vi "DAQFIFO_HH.vi"(0 "mode":u16(ring) items=["standalone", "dialog"]) -> ()   [LabVIEW 2009]
panel:
  in  "rebinning":dbl=16.0
  in  ".sm file format":bool
  in  "Exit":bool caption="stop"
  in  "Show Decay":bool=TRUE
  out "Counts":cluster{"Total":u32, "Gap":u32, "Invalid":u32}
  in  "Save & Exit":bool caption="stop"
  in  "Run":bool
  out "MCS":i32[][](graph)
  in  "Destination:":path
  in  "Store Data":bool caption="Store Data:"
  out "Decay":cluster{dbl[], u32[]}[](graph)
  out "SPC_rates":T1={"SYNC"=9999872.0, "Ch1"=44672.0, "Ch2"=44496.0, "Ch3"=44496.0, "Ch4"=44496.0, "Sync LED"=FALSE} {"Ch4" scale=1000.0..100000.0 scale format="%.0e"; "Ch3" scale=1000.0..100000.0 scale format="%.0e"; "Ch2" scale=1000.0..100000.0 scale format="%.0e"; "Ch1" min=0.0 max=8000000.0 scale=1.0..100000.0 scale format="%.0e"; "SYNC" min=0.0 max=100000000.0 scale=100000.0..100000000.0 scale format="%.0e"}
  in  "Tab Control":T2(tab)
  in  "Measurement":T3={"Binning (ms)"=1.0, "External Trigger Condition?"=0, "Stop Condition:"=2, "Stop Count"=120.0, "Buffer Size (Photons)?"=36864, "No of Channels?"=7, "Ext Latch Delay?"=0} {"Ext Latch Delay?" min=0 max=255 step=1; "Buffer Size (Photons)?" min=512 max=131072 step=512; "Stop Count" format="%.2f"; "Stop Condition:" items=["None", "Photon Count", "Time (s)"]; "No of Channels?" max=255 step=1; "Binning (ms)" min=1e-07 max=100000 format="%.3f"}
  in  "ADC":T4={"Binning (HH)"=1, "?Dither Range"=0, "?Count Increment"=1, "Mode"=1} {"Mode" items=["T3"]; "Binning (HH)" items=["1", "2", "4", "8", "16", "32", "64", "128", "256", "512", "1024"]; "?Count Increment" min=1 max=255 step=1; "?Dither Range" min=0 max=256 step=32}
  in  "SYNC":T5={"SYNC ZC Level (mV)"=10.0, "SYNC Freq Divider"=3, "SYNC Holdoff (ps)"=0.0, "SYNC Threshold (mV)"=200.0} {"SYNC Threshold (mV)" min=0 max=1000 format="%.2f"; "SYNC Holdoff (ps)" min=-99999 max=99999 format="%.2f"; "SYNC Freq Divider" items=["1", "2", "4", "8", "16"]; "SYNC ZC Level (mV)" min=0 max=40 format="%.2f"}
  in  "Ch1":T6={"Ch1 ZC Level (mV)"=10.0, "Ch1 Holdoff (ps)"=0.0, "Ch1 Threshold (mV)"=200.0} {"Ch1 Threshold (mV)" min=0 max=1000 format="%.2f"; "Ch1 Holdoff (ps)" min=-99999 max=99999 format="%.2f"; "Ch1 ZC Level (mV)" min=0 max=40 format="%.2f"}
  in  "Ch 2":T7={"Ch2 ZC Level (mV)"=10.0, "Ch2 Holdoff (ps)"=0.0, "Ch2 Threshold (mV)"=200.0} {"Ch2 Threshold (mV)" min=0 max=1000 format="%.2f"; "Ch2 Holdoff (ps)" min=-99999 max=99999 format="%.2f"; "Ch2 ZC Level (mV)" min=0 max=40 format="%.2f"}
  in  "Ch 3":T8={"Ch3 ZC Level (mV)"=10.0, "Ch3 Holdoff (ps)"=0.0, "Ch3 Threshold (mV)"=200.0} {"Ch3 Threshold (mV)" min=0 max=1000 format="%.2f"; "Ch3 Holdoff (ps)" min=-99999 max=99999 format="%.2f"; "Ch3 ZC Level (mV)" min=0 max=40 format="%.2f"}
  in  "Ch 4":T9={"Ch4 ZC Level (mV)"=10.0, "Ch4 Holdoff (ps)"=0.0, "Ch4 Threshold (mV)"=200.0} {"Ch4 Threshold (mV)" min=0 max=1000 format="%.2f"; "Ch4 Holdoff (ps)" min=-99999 max=99999 format="%.2f"; "Ch4 ZC Level (mV)" min=0 max=40 format="%.2f"}
  in  "TAC":T10={"TAC Range [ns]"=50.0, "TAC Gain"=2, "TAC Offset [%]"=0.0, "TAC Limit Low [%]"=0.0, "TAC Limit High [%]"=100.0} {"TAC Limit High [%]" min=0 max=100 format="%.2f"; "TAC Limit Low [%]" min=0 max=100 format="%.2f"; "TAC Offset [%]" min=0 max=100 format="%.2f"; "TAC Gain" min=1 max=15 step=1; "TAC Range [ns]" min=0 max=2000 format="%.2f"}
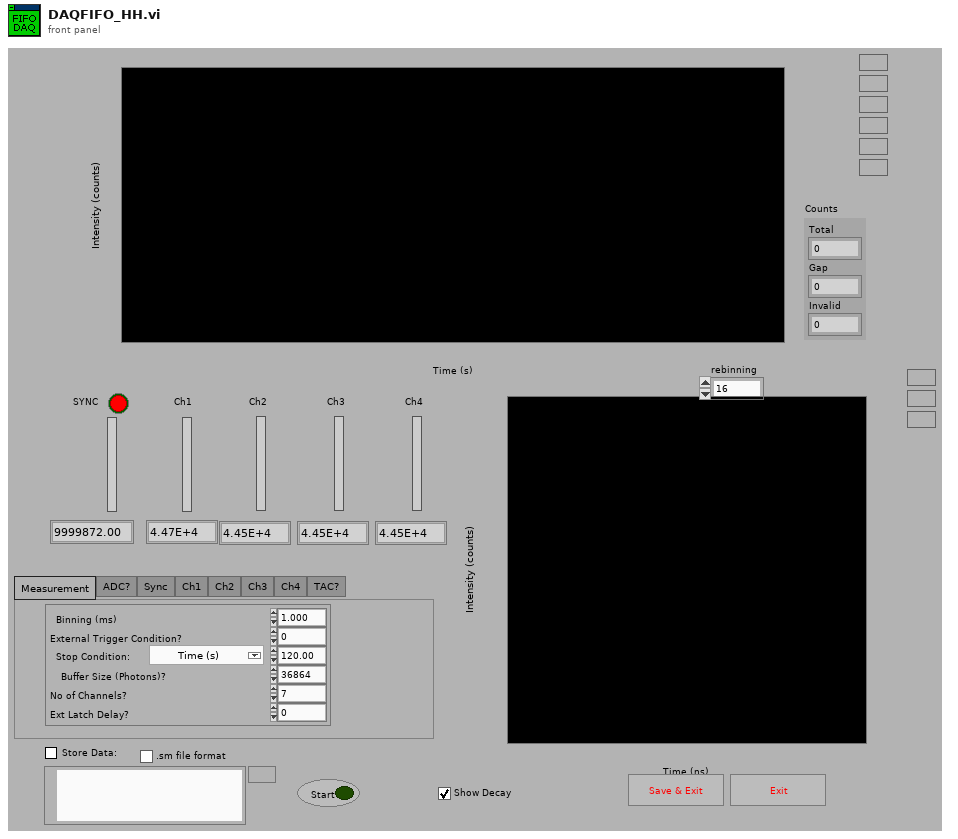
[diagram p1: front panel]
types:
  T1 = cluster{"SYNC":dbl, "Ch1":dbl, "Ch2":dbl, "Ch3":dbl, "Ch4":dbl, "Sync LED":bool}
  T2 = enum32{"Measurement", "ADC?", "Sync", "Ch1", "Ch2", "Ch3", "Ch4", "TAC?"}
  T3 = cluster{"Binning (ms)":sgl, "External Trigger Condition?":u16, "Stop Condition:":u16, "Stop Count":dbl, "Buffer Size (Photons)?":u32, "No of Channels?":u16, "Ext Latch Delay?":i16}
  T4 = cluster{"Binning (HH)":i16, "?Dither Range":i16, "?Count Increment":i16, "Mode":u16}
  T5 = cluster{"SYNC ZC Level (mV)":sgl, "SYNC Freq Divider":u16, "SYNC Holdoff (ps)":sgl, "SYNC Threshold (mV)":sgl}
  T6 = cluster{"Ch1 ZC Level (mV)":sgl, "Ch1 Holdoff (ps)":sgl, "Ch1 Threshold (mV)":sgl}
  T7 = cluster{"Ch2 ZC Level (mV)":sgl, "Ch2 Holdoff (ps)":sgl, "Ch2 Threshold (mV)":sgl}
  T8 = cluster{"Ch3 ZC Level (mV)":sgl, "Ch3 Holdoff (ps)":sgl, "Ch3 Threshold (mV)":sgl}
  T9 = cluster{"Ch4 ZC Level (mV)":sgl, "Ch4 Holdoff (ps)":sgl, "Ch4 Threshold (mV)":sgl}
  T10 = cluster{"TAC Range [ns]":sgl, "TAC Gain":i16, "TAC Offset [%]":sgl, "TAC Limit Low [%]":sgl, "TAC Limit High [%]":sgl}
  T11 = typedef "FIFOSettings.ctt" = cluster{"Measurement":cluster{"Binning (ms)":sgl, "External Trigger Condition":u16, "Stop Condition:":u16, "Stop Count":dbl, "Buffer Size (Photons)":u32, "No of Channels":u16, "Ext Latch Delay":i16}, "ADC":cluster{"Binning (HH)":i16, "Dither Range":i16, "Count Increment":i16, "Mode":u16}, "SYNC":cluster{"SYNC ZC Level (mV)":sgl, "SYNC Freq Divider":u16, "SYNC Holdoff (ps)":sgl, "SYNC Threshold (mV)":sgl}, "TAC":cluster{"TAC Range (ns)":sgl, "TAC Gain":i16, "TAC Offset (%)":sgl, "TAC Limit Low (%)":sgl, "TAC Limit High (%)":sgl}, "Ch 2":cluster{"Ch2 ZC Level (mV)":sgl, "Ch2 Holdoff (ps)":sgl, "Ch2 Threshold (mV)":sgl}, "Ch 3":cluster{"Ch3 ZC Level (mV)":sgl, "Ch3 Holdoff (ps)":sgl, "Ch3 Threshold (mV)":sgl}, "Ch 4":cluster{"Ch4 ZC Level (mV)":sgl, "Ch4 Holdoff (ps)":sgl, "Ch4 Threshold (mV)":sgl}, "Ch1":cluster{"Ch1 ZC Level (mV)":sgl, "Ch1 Holdoff (ps)":sgl, "Ch1 Threshold (mV)":sgl}}
  T12 = cluster{"Binning (ms)":sgl, "External Trigger Condition":u16, "Stop Condition:":u16, "Stop Count":dbl, "Buffer Size (Photons)":u32, "No of Channels":u16, "Ext Latch Delay":i16}
  T13 = cluster{"Binning (HH)":i16, "Dither Range":i16, "Count Increment":i16, "Mode":u16}
  T14 = cluster{"TAC Range (ns)":sgl, "TAC Gain":i16, "TAC Offset (%)":sgl, "TAC Limit Low (%)":sgl, "TAC Limit High (%)":sgl}
  T15 = cluster{"router channels":u8[], "macro times(50ns steps)":u32[], "micro times":u16[], "invalid times":u32[], "gap times":u32[]}
  T16 = cluster{"Sync_rate":sgl, "Ch1":sgl, "Ch2":sgl, "Ch3":sgl, "Ch 4":sgl, "Sync":bool}
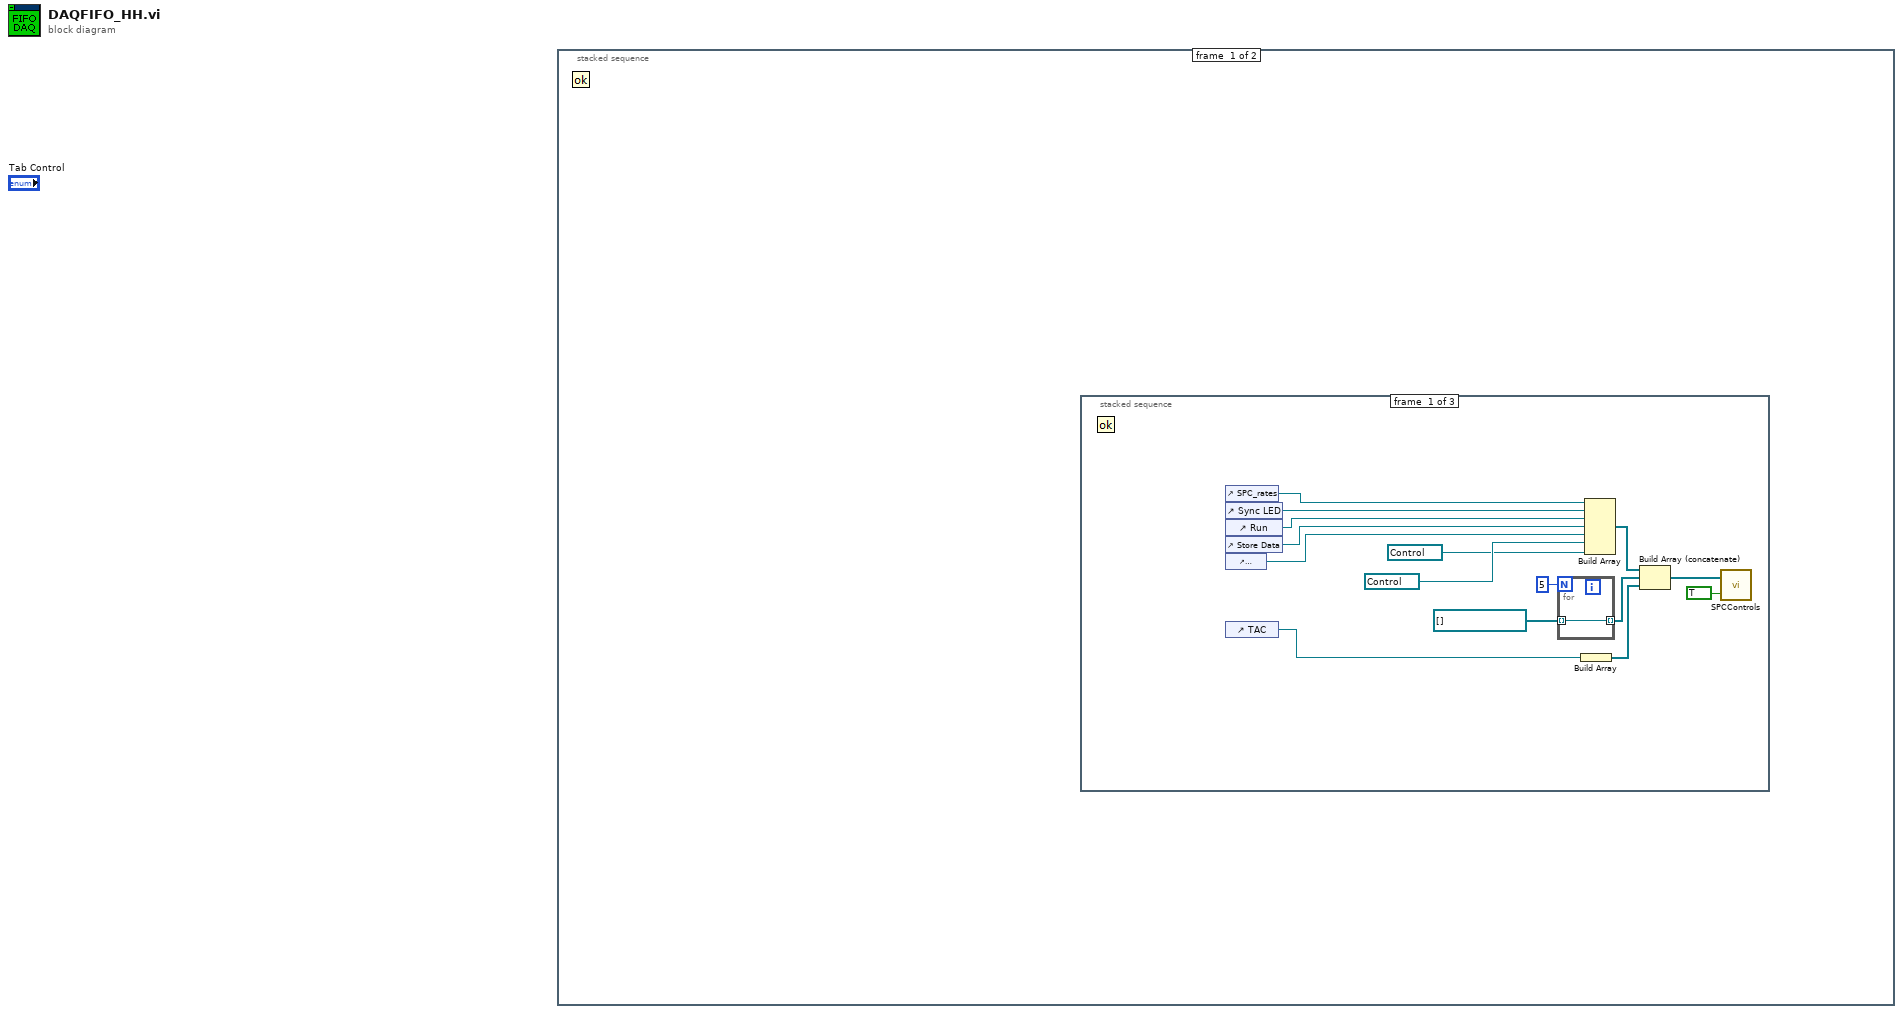
[diagram p0: block diagram]
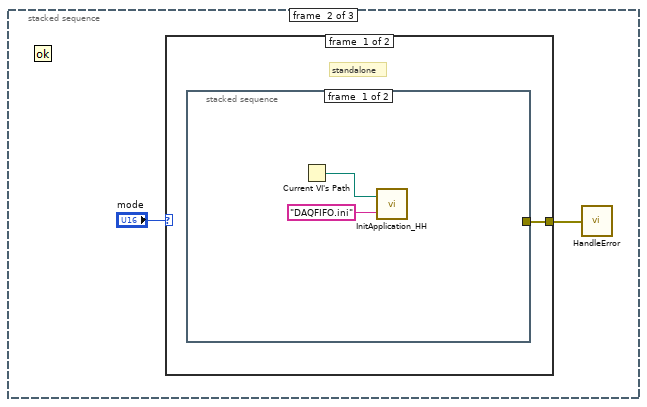
[diagram p2: hidden frame]
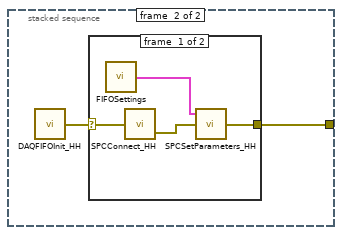
[diagram p3: hidden frame]
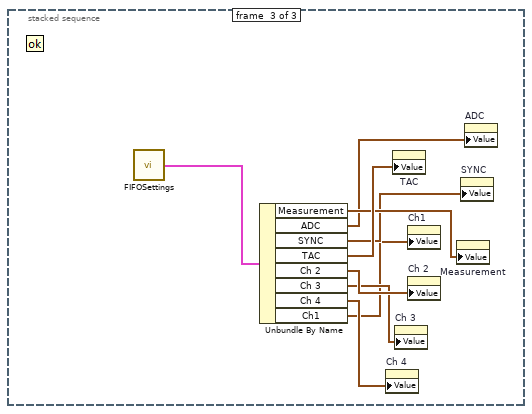
[diagram p6: hidden frame]
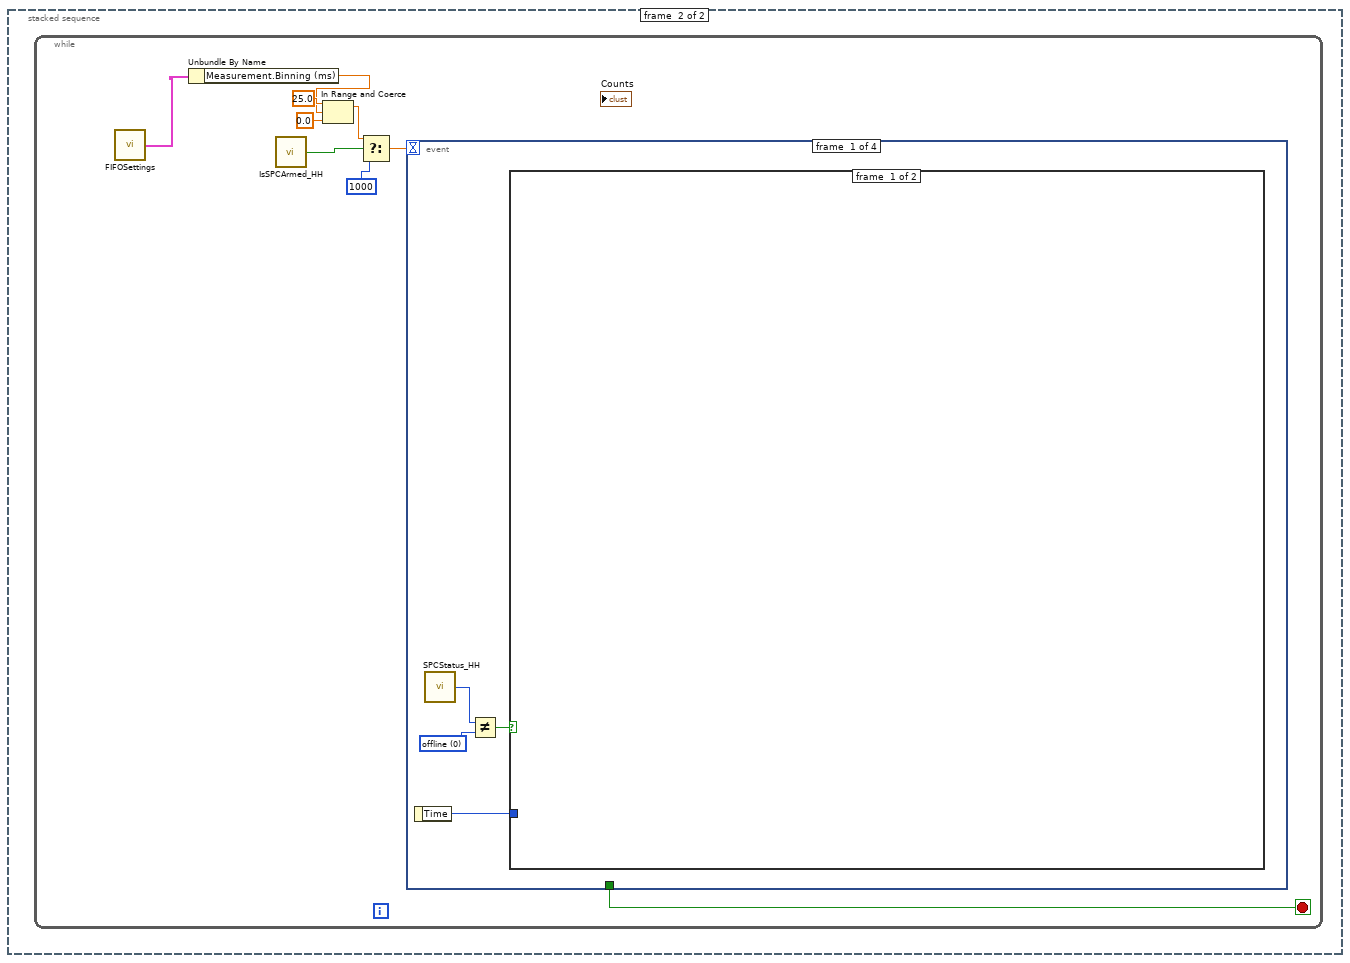
[diagram p7: hidden frame]
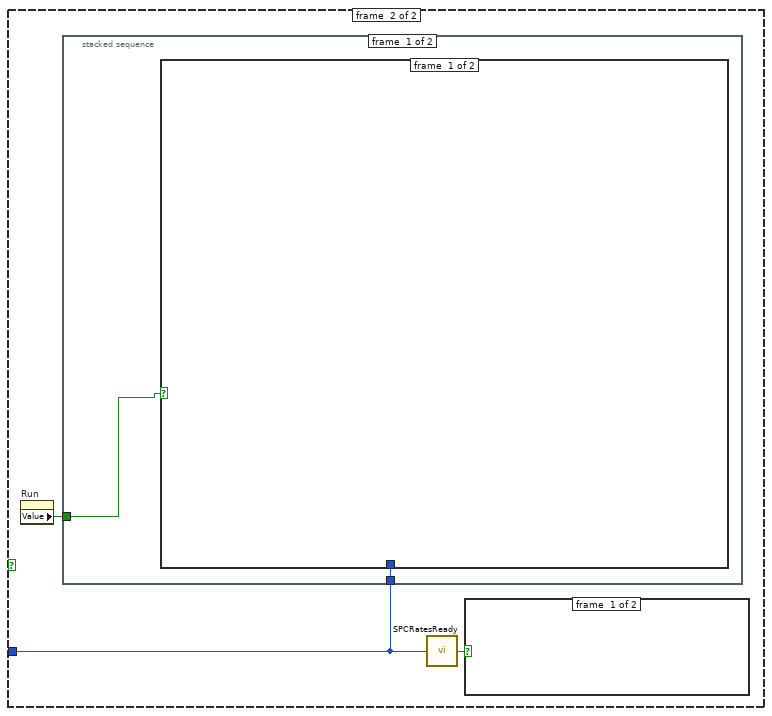
[diagram p8: hidden frame]
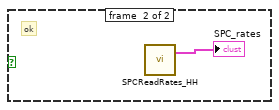
[diagram p9: hidden frame]
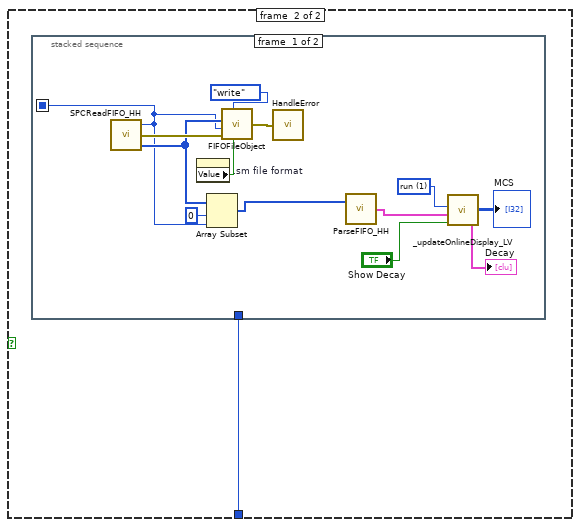
[diagram p10: hidden frame]
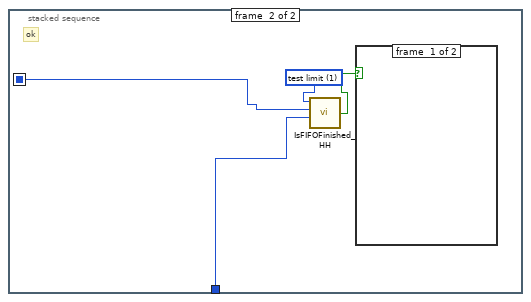
[diagram p11: hidden frame]
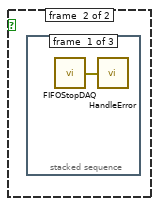
[diagram p12: hidden frame]
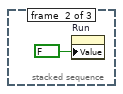
[diagram p13: hidden frame]
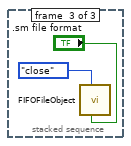
[diagram p14: hidden frame]
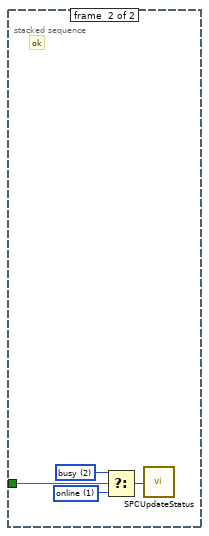
[diagram p15: hidden frame]
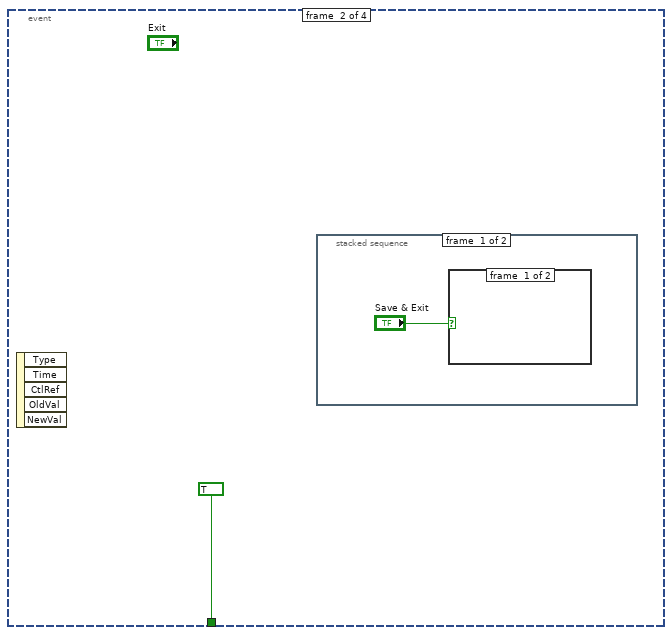
[diagram p16: hidden frame]
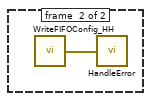
[diagram p17: hidden frame]
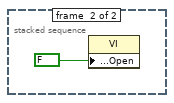
[diagram p18: hidden frame]
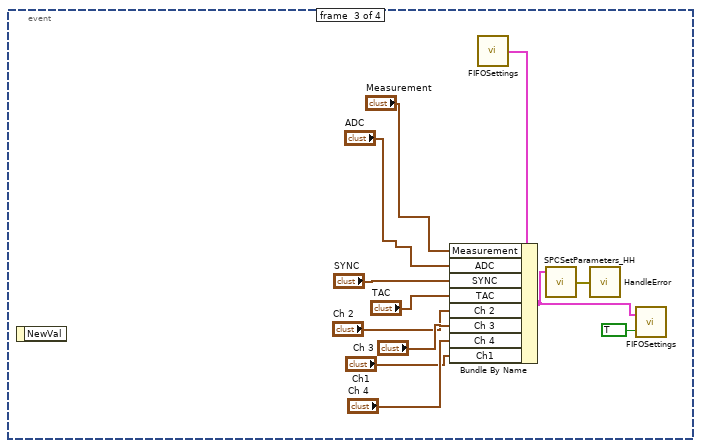
[diagram p19: hidden frame]
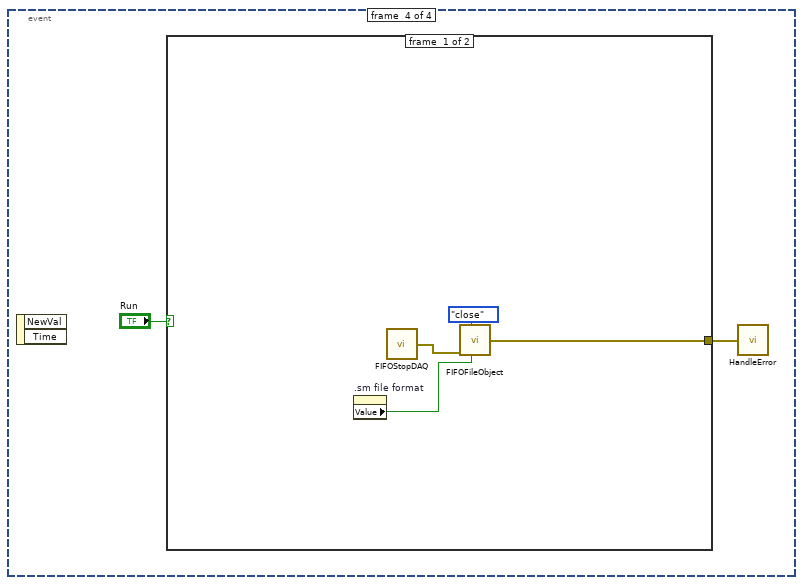
[diagram p20: hidden frame]
diagram:
  n1 = stacked-sequence {
    frame #0 {
      n2 = stacked-sequence {
        frame #0 {
          n3 = control-ref of="SPC_rates"() -> (w14:refnum<vi>)
          n4 = control-ref of="Sync LED"() -> (w13:refnum<vi>)
          n5 = control-ref of="Run"() -> (w8:refnum<vi>)
          n6 = control-ref of="Store Data"() -> (w9:refnum<vi>)
          n7 = control-ref of="Destination:"() -> (w10:refnum<vi>)
          n8 = control-ref of="TAC"() -> (w15:refnum<vi>)
          n9 = for {
            N: 5 -> [_]
            tunnel: refnum<vi>[] [] ("Controls[]") -> [w16] mode=indexing
            tunnel: [w16] -> w4 mode=indexing
          }
          n10 = Build Array(w15) -> (w12:refnum<vi>[])
          n11 = Build Array(w14, w13, w8, w9, w10, refnum<vi> refnum ("Element"), refnum<vi> refnum ("Element")) -> (w11:refnum<vi>[])
          n12 = Build Array (concatenate)(w11, w4, w12) -> (w7:refnum<vi>[])
          n13 = call "SPCControls.vi"("Set/Get"=TRUE, "Control References (input)"=w7) -> ()  [unwired: 1 out]
        }
        frame #1 {
          n14 = case shown="0, Default" "mode" {
            tunnel: [w19 _] -> w17
            frame #0 {
              # "standalone"
              n15 = stacked-sequence {
                tunnel: [_ w22] -> w19
                frame #0 {
                  n16 = Current VI's Path() -> (path=w21:path)
                  n17 = call "InitApplication_HH.vi"("file name"="DAQFIFO.ini" ("configuration file path"), "VI path"=w21) -> ()
                }
                frame #1 {
                  n18 = call "DAQFIFOInit_HH.vi"() -> ("error out"=w23:errorcluster)  [unwired: 1 in]
                  n19 = case shown="No Error" w23 {
                    selector: w23 -> [w27 w28]
                    tunnel: [w25 w28] -> w22
                    frame #0 {
                      n20 = call "FIFOSettings.vi"() -> ("FIFO Settings(out)"=w24:T11)  [unwired: 2 in]
                      n21 = call "SPCConnect_HH.vi"("error in (no error)"=w27) -> ("Error out"=w26:errorcluster)  [unwired: 1 in]
                      n22 = call "SPCSetParameters_HH.vi"("error in (no error)"=w26, "FIFO Settings"=w24) -> ("error (out)"=w25:errorcluster)  [unwired: 1 in]
                    }
                    frame #1 {
                    }
                  }
                }
              }
            }
            frame #1 {
              # "dialog"
            }
          }
          n23 = call "HandleError.vi"("error in (no error)"=w17) -> ()
        }
        frame #2 {
          n24 = call "FIFOSettings.vi"() -> ("FIFO Settings(out)"=w29:T11)  [unwired: 2 in]
          n25 = Unbundle By Name(w29) -> ("Measurement"=w36:T12, "ADC"=w35:T13, "SYNC"=w34:T5, "TAC"=w37:T14, "Ch 2"=w33:T7, "Ch 3"=w32:T8, "Ch 4"=w31:T9, "Ch1"=w30:T6)
          n26 = property on="Ch 4" class="Cluster (strikt)"("Value"=w31) -> ()  [unwired: 2 in, 2 out]
          n27 = property on="TAC" class="Cluster (strict)"("Value"=w37) -> ()  [unwired: 2 in, 2 out]
          n28 = property on="Ch 3" class="Cluster (strikt)"("Value"=w32) -> ()  [unwired: 2 in, 2 out]
          n29 = property on="Ch1" class="Cluster (strikt)"("Value"=w30) -> ()  [unwired: 2 in, 2 out]
          n30 = property on="Ch 2" class="Cluster (strikt)"("Value"=w33) -> ()  [unwired: 2 in, 2 out]
          n31 = property on="Measurement" class="Cluster (strikt)"("Value"=w36) -> ()  [unwired: 2 in, 2 out]
          n32 = property on="SYNC" class="Cluster (strikt)"("Value"=w34) -> ()  [unwired: 2 in, 2 out]
          n33 = property on="ADC" class="Cluster (strikt)"("Value"=w35) -> ()  [unwired: 2 in, 2 out]
        }
      }
    }
    frame #1 {
      n34 = while {
        stop <- w43 stop-if-true
        n35 = call "FIFOSettings.vi"() -> ("FIFO Settings(out)"=w38:T11)  [unwired: 2 in]
        n36 = Unbundle By Name(w38) -> ("Measurement.Binning (ms)"=w40:sgl)
        n37 = call "IsSPCArmed_HH.vi"() -> ("Boolean"=w46:bool)  [unwired: 1 in]
        n38 = In Range and Coerce(upper limit=25.0, x=w40, lower limit=0.0) -> (coerced(x)=w39:dbl)  [unwired: 1 out]
        n39 = Select(t=w39, s=w46, f=1000) -> (s? t:f=w44:dbl)
        n40 = event shown="[3] \"Run\": Value Change" {
          selector: _ -> [_ _ _ _]
          dyn-events: _ -> [_ _ _ _]
          timeout: w44 -> [_ _ _ _]
          tunnel: [_ TRUE _ _] -> w43
          event #0 {
            w50 = u16 0 items=["offline", "online", "busy"] ("Status")
            n41 = event-data() -> ("Time"=w47:u32)  [unwired: 1 in]
            n42 = call "SPCStatus_HH.vi"() -> ("Status (output)"=w48:enum16{"offline", "online", "busy"})  [unwired: 2 in]
            n43 = Not Equal?(x=w48, y=w50) -> (x != y?=w49:bool)
            n44 = case shown="True" w49 {
              tunnel: w47 -> [_ w53]
              frame #0 {
              }
              frame #1 {
                n45 = property on="Run" class="Boolean (strict)"() -> ("Value"=w52:bool)  [unwired: 2 in, 2 out]
                n46 = stacked-sequence {
                  tunnel: w52 -> [w55 w79]
                  tunnel: w53 -> [w56 _]
                  frame #0 {
                    n47 = case shown="True" w55 {
                      tunnel: w56 -> [_ w57]
                      frame #0 {
                      }
                      frame #1 {
                        n48 = stacked-sequence {
                          seq-local: [w65 _] -> [_ w71]
                          tunnel: w57 -> [_ w72]
                          frame #0 {
                            w62 = u16 1 items=["init", "run"] ("mode")
                            n49 = call "SPCReadFIFO_HH.vi"() -> ("count"=w65:i32, "error out"=w68:errorcluster, "buffer"=w66:u32[])  [unwired: 2 in]
                            n50 = property on=".sm file format" class="Bool (strict)"() -> ("Value"=w67:bool)  [unwired: 2 in, 2 out]
                            n51 = Array Subset(array=w66, index=0, length=w65) -> (w63:u32[])
                            n52 = call "FIFOFileObject.vi"(".sm file format"=w67, "function (open:0)"=enum16{"open", "write", "close"}."write", "error in (no error)"=w68, "count"=w65, "buffer"=w66) -> ("error out"=w70:errorcluster)  [unwired: 1 in]
                            n53 = call "HandleError.vi"("error in (no error)"=w70) -> ()
                            n54 = call "ParseFIFO_HH.vi"("RawData"=w63) -> ("RawData Out"=w59:T15)  [unwired: 1 in]
                            n55 = call "_updateOnlineDisplay_LV.vi"("show lifetime"="Show Decay", "Raw Data"=w59, "mode"=w62) -> ("lifetime histograms"=→"Decay":cluster{dbl[], u32[]}[], "Timetraces"=→"MCS":i32[][])  [unwired: 1 in]
                          }
                          frame #1 {
                            w74 = u16 1 items=["initialize", "test limit"] ("operation")
                            # "ok"
                            n56 = call "IsFIFOFinished_HH.vi"("Time"=w72, "Counts"=w71, "operation"=w74) -> ("Boolean"=w73:bool)  [unwired: 1 in]
                            n57 = case shown="True" w73 {
                              frame #0 {
                              }
                              frame #1 {
                                n58 = stacked-sequence {
                                frame #0 {
                                n59 = call "FIFOStopDAQ.vi"() -> ("error out"=w75:errorcluster)
                                n60 = call "HandleError.vi"("error in (no error)"=w75) -> ()
                                }
                                frame #1 {
                                n61 = property on="Run" class="Boolean (strict)"("Value"=FALSE ("Run")) -> ()  [unwired: 2 in, 2 out]
                                }
                                frame #2 {
                                n62 = call "FIFOFileObject.vi"(".sm file format"=".sm file format", "function (open:0)"=enum16{"open", "write", "close"}."close") -> ()  [unwired: 4 in, 1 out]
                                }
                                }
                              }
                            }
                          }
                        }
                      }
                    }
                  }
                  frame #1 {
                    w81 = u16 1 items=["offline", "online", "busy"] ("Status (input)")
                    w82 = u16 2 items=["offline", "online", "busy"] ("Status (input)")
                    # "ok"
                    n63 = Select(t=w82, s=w79, f=w81) -> (s? t:f=w80:u16)
                    n64 = call "SPCUpdateStatus.vi"("Status"=w80) -> ()
                  }
                }
                n65 = call "SPCRatesReady.vi"("Time"=w53) -> ("Boolean"=w51:bool)
                n66 = case shown="True" w51 {
                  frame #0 {
                  }
                  frame #1 {
                    # "ok"
                    n67 = call "SPCReadRates_HH.vi"() -> ("SPC_rates"=→"SPC_rates":T16)  [unwired: 1 out]
                  }
                }
              }
            }
          }
          event #1 {
            n68 = event-data() -> ()  [unwired: 1 in, 5 out]
            n69 = stacked-sequence {
              frame #0 {
                n70 = case shown="True" "Save & Exit" {
                  frame #0 {
                  }
                  frame #1 {
                    n71 = call "WriteFIFOConfig_HH.vi"() -> ("error out"=w85:errorcluster)  [unwired: 1 in]
                    n72 = call "HandleError.vi"("error in (no error)"=w85) -> ()
                  }
                }
              }
              frame #1 {
                n73 = property class="VI"("Front Panel Window:Open"=FALSE) -> ()  [unwired: 2 in, 2 out]
              }
            }
          }
          event #2 {
            n74 = event-data() -> ()  [unwired: 1 in, 1 out]
            n75 = call "FIFOSettings.vi"() -> ("FIFO Settings(out)"=w88:T11)  [unwired: 2 in]
            n76 = Bundle By Name(cluster=w88, "Measurement"="Measurement", "ADC"="ADC", "SYNC"="SYNC", "TAC"="TAC", "Ch 2"="Ch 2", "Ch 3"="Ch 3", "Ch 4"="Ch 4", "Ch1"="Ch1") -> (w87:T11)
            n77 = call "SPCSetParameters_HH.vi"("FIFO Settings"=w87) -> ("error (out)"=w91:errorcluster)  [unwired: 2 in]
            n78 = call "HandleError.vi"("error in (no error)"=w91) -> ()
            n79 = call "FIFOSettings.vi"("Set/Get"=TRUE, "FIFO Settings(in)"=w87) -> ()  [unwired: 1 out]
          }
          event #3 {
            n80 = event-data() -> ()  [unwired: 1 in, 2 out]
            n81 = case shown="True" "Run" {
              tunnel: [w102 w105] -> w100
              frame #0 {
                n82 = property on=".sm file format" class="Bool (strict)"() -> ("Value"=w101:bool)  [unwired: 2 in, 2 out]
                n83 = call "FIFOStopDAQ.vi"() -> ("error out"=w103:errorcluster)
                n84 = call "FIFOFileObject.vi"(".sm file format"=w101, "function (open:0)"=enum16{"open", "write", "close"}."close", "error in (no error)"=w103) -> ("error out"=w102:errorcluster)  [unwired: 3 in]
              }
              frame #1 {
                n85 = stacked-sequence {
                  seq-local: [w115 _] -> [_ w126]
                  tunnel: [_ w125] -> w105
                  frame #0 {
                    w109 = u16 0 items=["init", "run"] ("mode")
                    w107 = u16 0 items=["initialize", "test limit"] ("operation")
                    # "ok"
                    n86 = call "FIFOSettings.vi"() -> ("FIFO Settings(out)"=w110:T11)  [unwired: 2 in]
                    n87 = case shown="True" "Store Data" {
                      tunnel: [_ w123] -> w115
                      frame #0 {
                      }
                      frame #1 {
                        # "ok"
                        n88 = property on=".sm file format" class="Bool (strict)"() -> (error out=w120:errorcluster, "Value"=w119:bool)  [unwired: 2 in, 1 out]
                        n89 = call "WriteFIFOHeader_HH.vi"("error in"=w120, "Destination:"="Destination:") -> ("error out"=w121:errorcluster)
                        n90 = call "FIFOFileObject.vi"(".sm file format"=w119, "function (open:0)"=enum16{"open", "write", "close"}."open", "error in (no error)"=w121, "Destination:"="Destination:") -> ("error out"=w123:errorcluster)  [unwired: 2 in]
                      }
                    }
                    n91 = Unbundle By Name(w110) -> ("Measurement"=w112:T12, "Measurement.Stop Condition:"=w113:u16)
                    n92 = call "FIFOInitDAQ_HH.vi"() -> ()  [unwired: 1 in]
                    n93 = case shown="0, Default" w113 {
                      tunnel: [_ u32 0 ("Start (input)") w118] -> w111
                      frame #0 {
                      }
                      frame #1 {
                      }
                      frame #2 {
                        n94 = Tick Count (ms)() -> (millisecond timer value=w118:u32)
                      }
                    }
                    n95 = property on="Show Decay" class="Bool (strict)"() -> ("Value"=w108:bool)  [unwired: 2 in, 2 out]
                    n96 = call "_updateOnlineDisplay_LV.vi"("show lifetime"=w108, "mode"=w109, "rebinning"="rebinning") -> ()  [unwired: 1 in, 2 out]
                    n97 = call "IsFIFOFinished_HH.vi"("Measurement"=w112, "Time"=w111, "Counts"=w111, "operation"=w107) -> ()  [unwired: 1 out]
                    n98 = call "FIFOStart.vi"("Set/Get"=TRUE, "Start (input)"=w111) -> ()  [unwired: 1 out]
                  }
                  frame #1 {
                    n99 = case shown="No Error" w126 {
                      selector: w126 -> [w128 w133]
                      tunnel: [w129 w133] -> w125
                      frame #0 {
                        n100 = call "FIFOStartDAQ_HH.vi"("error in (no error)"=w128) -> ("error out"=w130:errorcluster)
                        n101 = case shown="No Error" w130 {
                          selector: w130 -> [_ w132]
                          tunnel: [_ w132] -> w129
                          frame #0 {
                            w131 = u16 2 items=["offline", "online", "busy"] ("Status (input)")
                            n102 = call "SPCUpdateStatus.vi"("Status"=w131) -> ()
                          }
                          frame #1 {
                          }
                        }
                      }
                      frame #1 {
                      }
                    }
                    n103 = case shown="No Error" w125 {
                      frame #0 {
                      }
                      frame #1 {
                        n104 = property on="Run" class="Boolean (strict)"("Value"=FALSE ("Run")) -> ()  [unwired: 2 in, 2 out]
                      }
                    }
                  }
                }
              }
            }
            n105 = call "HandleError.vi"("error in (no error)"=w100) -> ()
          }
        }
      }
    }
  }
